vi "load_conf_data.vi"(0 "file":path, 5 "SET Shunt":bool, 9 "SET Compensation":bool) -> (6 "Comp":cdb[](array[numeric]), 10 "Shunt":cdb[](array[numeric]))   [LabVIEW 2017, in "ZBOX_IS.lvlib"]
uses:
  ZBOX_IS.lvlib
  <vilib>/Utility/file.llb/Read From Spreadsheet File (DBL).vi
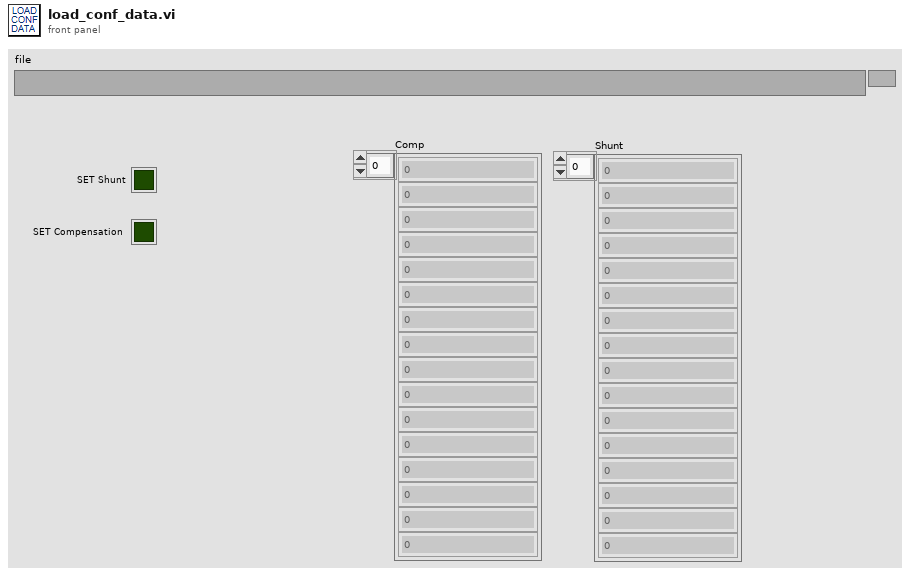
[diagram p1: front panel]
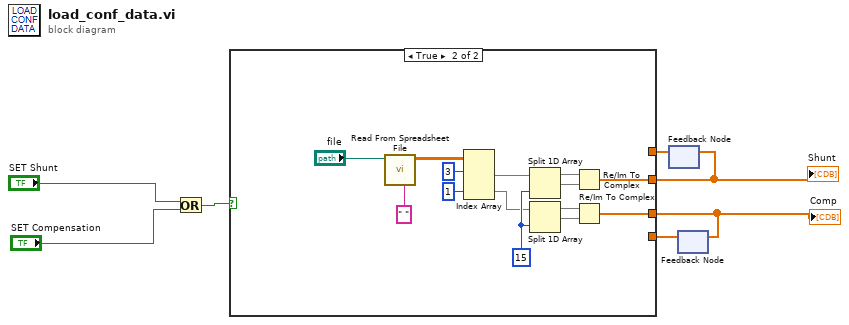
[diagram p0: block diagram]
diagram:
  n1 = Or(x="SET Shunt", y="SET Compensation") -> (x .or. y?=w3:bool)
  n2 = feedback #1() -> (w7:cdb[])  [unwired: 1 in]
  n3 = feedback #2() -> (w6:cdb[])  [unwired: 1 in]
  n4 = case shown="True" w3 {
    tunnel: [w9 w16] -> w2
    tunnel: [w8 w15] -> w1
    tunnel: w7 -> [w9 _]
    tunnel: w6 -> [w8 _]
    frame False {
    }
    frame True {
      w12 = 15 ("index")
      n5 = call-poly <vilib>:"Read From Spreadsheet File.vi"("delimiter (\\t)"=" " ("delimiter (\\t)"), "file path (dialog if empty)"="file") -> ("all rows"=w21:dbl[][])  [unwired: 5 in, 4 out]
      n6 = Index Array(array=w21, index (row) #1=3 ("index (row)"), index (row) #2=1 ("index (row)")) -> (element #1=w19:dbl[], element #2=w11:dbl[])  [unwired: 2 in]
      n7 = Split 1D Array(array=w19, index=w12) -> (first subarray=w18:dbl[], second subarray=w17:dbl[])
      n8 = Split 1D Array(array=w11, index=w12) -> (first subarray=w13:dbl[], second subarray=w14:dbl[])
      n9 = Re/Im To Complex(1:w17, 2:w18) -> (0:w16:cdb[])
      n10 = Re/Im To Complex(1:w14, 2:w13) -> (0:w15:cdb[])
    }
  }
  "Comp" <- w1
  "Shunt" <- w2
  n11 = feedback-in #1(w2) -> ()
  n12 = feedback-in #2(w1) -> ()
